vi "DROPBEAR_Model_Updating_Initialize.vi"(8 "error in (no error)":errorcluster, 11 "DROPBEAR_Model_Updating in":refnum<class "DROPBEAR_Model_Updating.lvclass">) -> (0 "error out":errorcluster, 3 "DROPBEAR_Model_Updating out":refnum<class "DROPBEAR_Model_Updating.lvclass">)   [LabVIEW 2021, in "DROPBEAR_Model_Updating.lvclass"]
uses:
  DROPBEAR_Model_Updating.lvclass
  DROPBEAR_Model_Updating.lvclass/DROPBEAR_Model_Updating.ctl
  Kalman_Filter/Kalman_Filter.lvclass
  FEA_Model/FEA_Model.lvclass
  MOCKBEAR/MOCKBEAR.lvclass
  Data_Array/Data_Array.lvclass
  Moving_Statistic/Moving_Statistic.lvclass
  Online_Statistic/Online_Statistic.lvclass
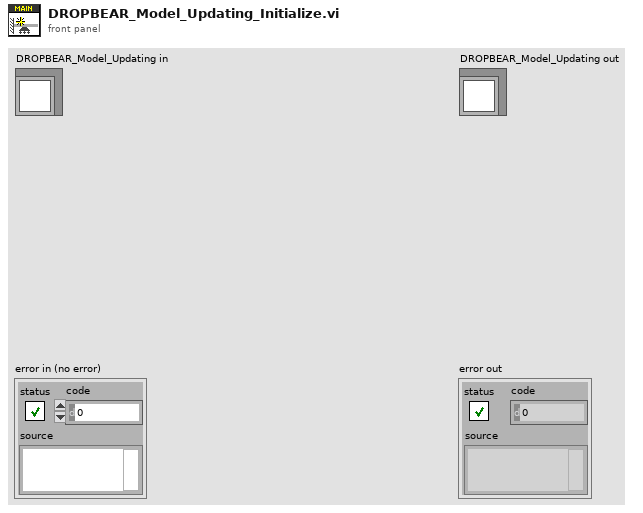
[diagram p1: front panel]
types:
  T1 = cluster{"Measurement Variance":dbl, "State Variance":dbl, "Threshold":dbl}
  T2 = cluster{"Frequency State":refnum<class "Kalman_Filter.lvclass">, "Rolling Condition State":refnum<class "Kalman_Filter.lvclass">, "Frequency State":dbl, "Pinned Condition State":dbl}
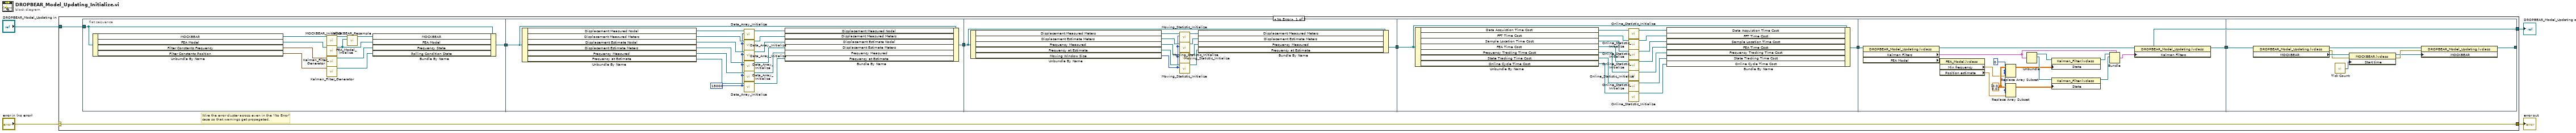
[diagram p0: block diagram]
diagram:
  n1 = case shown="No Error" "error in (no error)" {
    selector: "error in (no error)" -> [w12 w91]
    tunnel: [w12 w91] -> w3
    tunnel: [w7 w90] -> w1
    tunnel: "DROPBEAR_Model_Updating in" -> [w8 w90]
    frame No Error {
      # "Wire the error cluster across even in the \"No Error\"\ncase so that warnings get propagated."
      n2 = flat-sequence {
        tunnel: w8 -> [w17]
        tunnel: [w18] -> w11
        tunnel: w11 -> [w32]
        tunnel: [w25] -> w10
        tunnel: w10 -> [w44]
        tunnel: [w39] -> w9
        tunnel: w9 -> [w58]
        tunnel: [w50] -> w6
        tunnel: w6 -> [w81]
        tunnel: [w66] -> w5
        tunnel: [w82] -> w7
        tunnel: w5 -> [w89]
        frame #0 {
          n3 = Unbundle By Name(w17) -> ("MOCKBEAR"=w22:refnum<class "MOCKBEAR.lvclass">, "FEA Model"=w23:refnum<class "FEA_Model.lvclass">, "Filter Constants Frequency"=w14:T1, "Filter Constants Position"=w13:T1)
          n4 = call-dynamic "MOCKBEAR_Initialize.vi"("MOCKBEAR in"=w22) -> ("MOCKBEAR out"=w21:refnum<class "MOCKBEAR.lvclass">)  [unwired: 9 in, 1 out]
          n5 = call-dynamic "FEA_Model_Intialize.vi"("FEA_Model in"=w23) -> ("FEA_Model out"=w19:refnum<class "FEA_Model.lvclass">)  [unwired: 9 in, 1 out]
          n6 = call "Kalman_Filter_Generator.vi"("Filter Constants"=w14) -> ("Kalman_Filter out"=w16:refnum<class "Kalman_Filter.lvclass">)  [unwired: 9 in, 1 out]
          n7 = call "Kalman_Filter_Generator.vi"("Filter Constants"=w13) -> ("Kalman_Filter out"=w15:refnum<class "Kalman_Filter.lvclass">)  [unwired: 9 in, 1 out]
          n8 = call-dynamic "MOCKBEAR_Resample.vi"("FEA_Model in"=w19, "MOCKBEAR in"=w21) -> ("MOCKBEAR out"=w20:refnum<class "MOCKBEAR.lvclass">)  [unwired: 8 in, 1 out]
          n9 = Bundle By Name(cluster=w17, "MOCKBEAR"=w20, "FEA Model"=w19, "Frequency State"=w16, "Rolling Condition State"=w15) -> (w18:refnum<class "DROPBEAR_Model_Updating.lvclass">)
        }
        frame #1 {
          w24 = 15000
          n10 = Unbundle By Name(w32) -> ("Displacement Measured Nodal"=w38:refnum<class "Data_Array.lvclass">, "Displacement Measured Meters"=w37:refnum<class "Data_Array.lvclass">, "Displacement Estimate Nodal"=w36:refnum<class "Data_Array.lvclass">, "Displacement Estimate Meters"=w35:refnum<class "Data_Array.lvclass">, "Frequency Measured"=w34:refnum<class "Data_Array.lvclass">, "Frequency at Estimate"=w33:refnum<class "Data_Array.lvclass">)
          n11 = call-dynamic "Data_Array_Initialize.vi"("Buffer"=w24, "Data_Array in"=w38) -> ("Data_Array out"=w31:refnum<class "Data_Array.lvclass">)  [unwired: 8 in, 1 out]
          n12 = call-dynamic "Data_Array_Initialize.vi"("Buffer"=w24, "Data_Array in"=w37) -> ("Data_Array out"=w30:refnum<class "Data_Array.lvclass">)  [unwired: 8 in, 1 out]
          n13 = call-dynamic "Data_Array_Initialize.vi"("Buffer"=w24, "Data_Array in"=w36) -> ("Data_Array out"=w29:refnum<class "Data_Array.lvclass">)  [unwired: 8 in, 1 out]
          n14 = call-dynamic "Data_Array_Initialize.vi"("Buffer"=w24, "Data_Array in"=w35) -> ("Data_Array out"=w28:refnum<class "Data_Array.lvclass">)  [unwired: 8 in, 1 out]
          n15 = call-dynamic "Data_Array_Initialize.vi"("Buffer"=w24, "Data_Array in"=w34) -> ("Data_Array out"=w27:refnum<class "Data_Array.lvclass">)  [unwired: 8 in, 1 out]
          n16 = call-dynamic "Data_Array_Initialize.vi"("Buffer"=w24, "Data_Array in"=w33) -> ("Data_Array out"=w26:refnum<class "Data_Array.lvclass">)  [unwired: 8 in, 1 out]
          n17 = Bundle By Name(cluster=w32, "Displacement Measured Nodal"=w31, "Displacement Measured Meters"=w30, "Displacement Estimate Nodal"=w29, "Displacement Estimate Meters"=w28, "Frequency Measured"=w27, "Frequency at Estimate"=w26) -> (w25:refnum<class "DROPBEAR_Model_Updating.lvclass">)
        }
        frame #2 {
          n18 = Unbundle By Name(w44) -> ("Displacement Measured Meters"=w49:refnum<class "Moving_Statistic.lvclass">, "Displacement Estimate Meters"=w48:refnum<class "Moving_Statistic.lvclass">, "Frequency Measured"=w47:refnum<class "Moving_Statistic.lvclass">, "Frequency at Estimate"=w46:refnum<class "Moving_Statistic.lvclass">, "Moving Window Size"=w45:i32)
          n19 = call-dynamic "Moving_Statistic_Initialize.vi"("Window"=w45, "Moving_Mean in"=w49) -> ("Moving_Mean out"=w43:refnum<class "Moving_Statistic.lvclass">)  [unwired: 8 in, 1 out]
          n20 = call-dynamic "Moving_Statistic_Initialize.vi"("Window"=w45, "Moving_Mean in"=w48) -> ("Moving_Mean out"=w42:refnum<class "Moving_Statistic.lvclass">)  [unwired: 8 in, 1 out]
          n21 = call-dynamic "Moving_Statistic_Initialize.vi"("Window"=w45, "Moving_Mean in"=w47) -> ("Moving_Mean out"=w41:refnum<class "Moving_Statistic.lvclass">)  [unwired: 8 in, 1 out]
          n22 = call-dynamic "Moving_Statistic_Initialize.vi"("Window"=w45, "Moving_Mean in"=w46) -> ("Moving_Mean out"=w40:refnum<class "Moving_Statistic.lvclass">)  [unwired: 8 in, 1 out]
          n23 = Bundle By Name(cluster=w44, "Displacement Measured Meters"=w43, "Displacement Estimate Meters"=w42, "Frequency Measured"=w41, "Frequency at Estimate"=w40) -> (w39:refnum<class "DROPBEAR_Model_Updating.lvclass">)
        }
        frame #3 {
          n24 = Unbundle By Name(w58) -> ("Data Acquistion Time Cost"=w65:refnum<class "Online_Statistic.lvclass">, "FFT Time Cost"=w64:refnum<class "Online_Statistic.lvclass">, "Sample Location Time Cost"=w63:refnum<class "Online_Statistic.lvclass">, "FEA Time Cost"=w62:refnum<class "Online_Statistic.lvclass">, "Frequency Tracking Time Cost"=w61:refnum<class "Online_Statistic.lvclass">, "State Tracking Time Cost"=w60:refnum<class "Online_Statistic.lvclass">, "Online Cycle Time Cost"=w59:refnum<class "Online_Statistic.lvclass">)
          n25 = call-dynamic "Online_Statistic_Initialize.vi"("Online_Statistic in"=w65) -> ("Online_Statistic out"=w57:refnum<class "Online_Statistic.lvclass">)  [unwired: 9 in, 1 out]
          n26 = call-dynamic "Online_Statistic_Initialize.vi"("Online_Statistic in"=w64) -> ("Online_Statistic out"=w56:refnum<class "Online_Statistic.lvclass">)  [unwired: 9 in, 1 out]
          n27 = call-dynamic "Online_Statistic_Initialize.vi"("Online_Statistic in"=w63) -> ("Online_Statistic out"=w55:refnum<class "Online_Statistic.lvclass">)  [unwired: 9 in, 1 out]
          n28 = call-dynamic "Online_Statistic_Initialize.vi"("Online_Statistic in"=w62) -> ("Online_Statistic out"=w54:refnum<class "Online_Statistic.lvclass">)  [unwired: 9 in, 1 out]
          n29 = call-dynamic "Online_Statistic_Initialize.vi"("Online_Statistic in"=w61) -> ("Online_Statistic out"=w53:refnum<class "Online_Statistic.lvclass">)  [unwired: 9 in, 1 out]
          n30 = call-dynamic "Online_Statistic_Initialize.vi"("Online_Statistic in"=w60) -> ("Online_Statistic out"=w52:refnum<class "Online_Statistic.lvclass">)  [unwired: 9 in, 1 out]
          n31 = call-dynamic "Online_Statistic_Initialize.vi"("Online_Statistic in"=w59) -> ("Online_Statistic out"=w51:refnum<class "Online_Statistic.lvclass">)  [unwired: 9 in, 1 out]
          n32 = Bundle By Name(cluster=w58, "Data Acquistion Time Cost"=w57, "FFT Time Cost"=w56, "Sample Location Time Cost"=w55, "FEA Time Cost"=w54, "Frequency Tracking Time Cost"=w53, "State Tracking Time Cost"=w52, "Online Cycle Time Cost"=w51) -> (w50:refnum<class "DROPBEAR_Model_Updating.lvclass">)
        }
        frame #4 {
          w67 = 0 ("disabled index (col)")
          w72 = dbl[][] [[0.0], [0.0]] ("array")
          n33 = property class="DROPBEAR_Model_Updating.lvclass"(reference=w81) -> (reference out=w78:refnum<class "DROPBEAR_Model_Updating.lvclass">, "Kalman Filters"=w77:T2, "FEA Model"=w73:refnum<class "FEA_Model.lvclass">)  [unwired: 1 in, 1 out]
          n34 = property class="FEA_Model.lvclass"(reference=w73) -> ("Min frequency"=w69:dbl, "Position estimate"=w68:dbl)  [unwired: 1 in, 2 out]
          n35 = Replace Array Subset(array=w72, new element=w69, index (row)=w67, index (col)=w67) -> (w71:dbl[][])
          n36 = Replace Array Subset(array=w72, new element=w68, index (row)=w67, index (col)=w67) -> (w70:dbl[][])
          n37 = Unbundle(w77) -> ("Frequency State"=w80:refnum<class "Kalman_Filter.lvclass">, "Rolling Condition State"=w79:refnum<class "Kalman_Filter.lvclass">)  [unwired: 2 out]
          n38 = property class="Kalman_Filter.lvclass"(reference=w80, "State"=w71) -> (reference out=w75:refnum<class "Kalman_Filter.lvclass">)  [unwired: 1 in, 1 out]
          n39 = property class="Kalman_Filter.lvclass"(reference=w79, "State"=w70) -> (reference out=w74:refnum<class "Kalman_Filter.lvclass">)  [unwired: 1 in, 1 out]
          n40 = Bundle(cluster=w77, "Frequency State"=w75, "Rolling Condition State"=w74) -> (w76:T2)  [unwired: 2 in]
          n41 = property class="DROPBEAR_Model_Updating.lvclass"(reference=w78, "Kalman Filters"=w76) -> (reference out=w66:refnum<class "DROPBEAR_Model_Updating.lvclass">)  [unwired: 1 in, 1 out]
        }
        frame #5 {
          n42 = property class="DROPBEAR_Model_Updating.lvclass"(reference=w89) -> (reference out=w83:refnum<class "DROPBEAR_Model_Updating.lvclass">, error out=w86:errorcluster, "MOCKBEAR"=w88:refnum<class "MOCKBEAR.lvclass">)  [unwired: 1 in]
          n43 = call "Tick Count"() -> ("Tick Count(uSec)"=w87:u32)
          n44 = property class="MOCKBEAR.lvclass"(reference=w88, error in=w86, "Start time"=w87) -> (reference out=w84:refnum<class "MOCKBEAR.lvclass">, error out=w85:errorcluster)
          n45 = property class="DROPBEAR_Model_Updating.lvclass"(reference=w83, error in=w85, "MOCKBEAR"=w84) -> (reference out=w82:refnum<class "DROPBEAR_Model_Updating.lvclass">)  [unwired: 1 out]
        }
      }
    }
    frame Error {
    }
  }
  "error out" <- w3
  "DROPBEAR_Model_Updating out" <- w1
